vi "decode varint.vi"(10 "read index in":i32, 11 "byte array in":u8[](array[numeric]) format="%.0b") -> (1 "value":u64, 2 "read index out":i32)   [LabVIEW 2013, in "protocol buffers encoder.lvlib"]
uses:
  protocol buffers encoder.lvlib
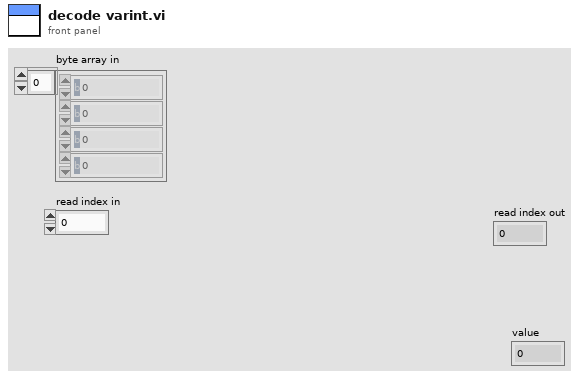
[diagram p1: front panel]
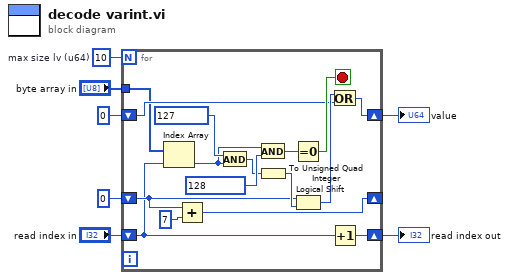
[diagram p0: block diagram]
diagram:
  w7 = 10  # max size lv (u64)
  n1 = for {
    N: w7 -> [_]
    tunnel: "byte array in" -> [w11]
    shift-right: [w19] -> w4
    shift-left: u64 0 -> [w12]
    shift-right: [w14] -> _
    shift-left: u64 0 -> [w13]
    shift-right: [w8] -> w1
    shift-left: "read index in" -> [w9]
    stop <- w22 stop-if-true
    n2 = Index Array(array=w11, index=w9) -> (element=w10:u8)
    n3 = Add(x=w13, y=u64 7) -> (x+y=w14:u64)
    n4 = And(x=u8 127 ("y"), y=w10) -> (x .and. y?=w18:u8)
    n5 = And(x=w10, y=u8 128) -> (x .and. y?=w23:u8)
    n6 = To Unsigned Quad Integer(1:w18) -> (0:w17:u64)
    n7 = Equal To 0?(x=w23) -> (x = 0?=w22:bool)
    n8 = Logical Shift(y=w13, x=w17) -> (x << y=w16:u64)
    n9 = Or(x=w16, y=w12) -> (x .or. y?=w19:u64)
    n10 = Increment(x=w9) -> (x+1=w8:i32)
  }
  "value" <- w4
  "read index out" <- w1
